vi "ExecuteCommand.vi"(11 "Command":string) -> ()   [LabVIEW 2015]
uses:
  <vilib>/Rock Robotics/Network Tables/SD Write String.vi
panel:
  out "array w/ subset deleted":string[](array[string])
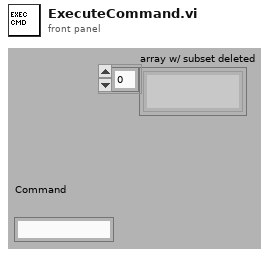
[diagram p1: front panel]
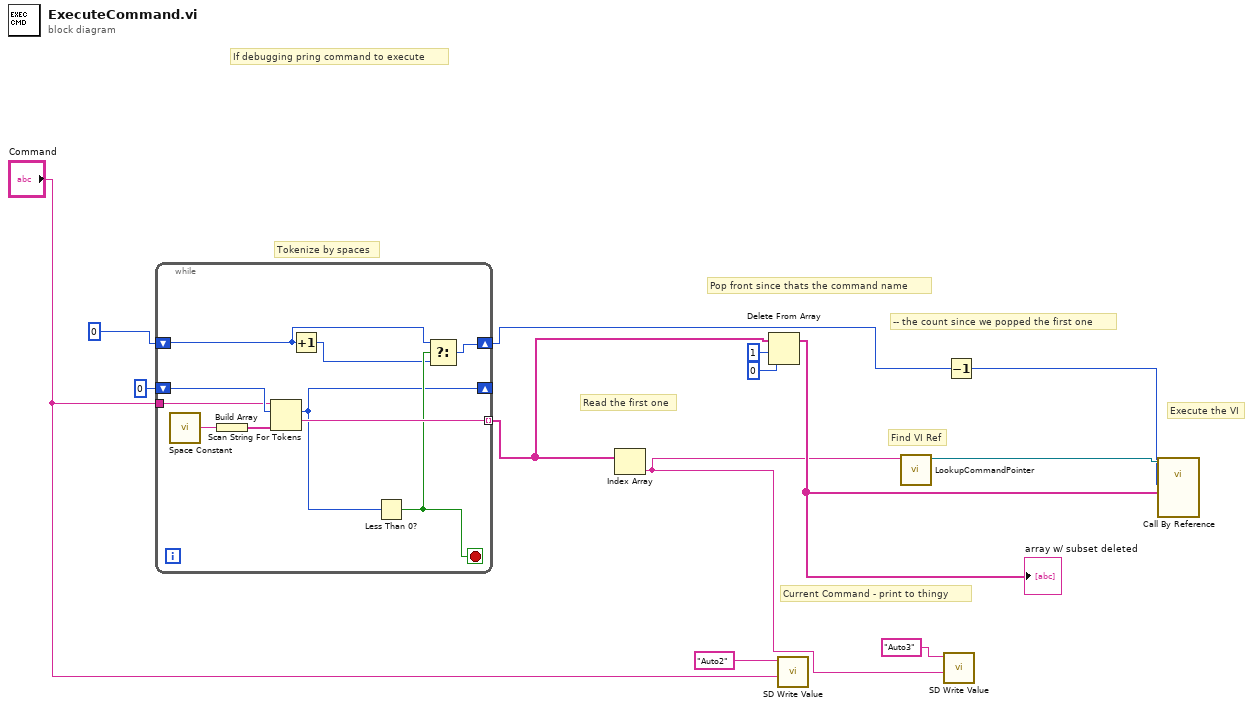
[diagram p0: block diagram]
diagram:
  # "Current Command - print to thingy"
  # "If debugging pring command to execute"
  # "Execute the VI"
  # "-- the count since we popped the first one"
  # "Pop front since thats the command name"
  # "Find VI Ref"
  # "Read the first one"
  # "Tokenize by spaces"
  n1 = while {
    shift-right: [w14] -> _
    shift-left: 0 ("offset past token") -> [w23]
    tunnel: "Command" -> [w22]
    tunnel: [w21] -> w7 mode=indexing
    shift-right: [w17] -> w10
    shift-left: u8 0 -> [w19]
    stop <- w20 stop-if-true
    n2 = call <vilib>:"Space Constant.vi"() -> ("String"=w16:string)
    n3 = Build Array(w16) -> (w15:string[])
    n4 = Scan String For Tokens(6:w15, 8:w23, 9:w22) -> (1:w21:string, 2:w14:i32)  [unwired: 5 out]
    n5 = Increment(x=w19) -> (x+1=w18:u8)
    n6 = Less Than 0?(x=w14) -> (x < 0?=w20:bool)
    n7 = Select(t=w19, s=w20, f=w18) -> (s? t:f=w17:u8)
  }
  n8 = Index Array(array=w7) -> (element=w3:string)  [unwired: 1 in]
  n9 = Delete From Array(array=w7, length=1, index=0) -> (array with subset deleted=w5:string[])  [unwired: 1 out]
  "array w/ subset deleted" <- w5
  n10 = call-poly <vilib>:"SD Write Value.vi"("String"="Command", "Name"="Auto2") -> ()  [unwired: 8 in, 2 out]
  n11 = call "LookupCommandPointer.vi"("refnum name"=w3) -> ("VI Refnum Out"=w9:refnum<vi>)  [unwired: 10 out]
  n12 = call-poly <vilib>:"SD Write Value.vi"("String"=w3, "Name"="Auto3") -> ()  [unwired: 8 in, 2 out]
  n13 = Decrement(x=w10) -> (x-1=w8:u8)
  n14 = call-by-ref "?"(reference=w9, "argv"=w5, "args"=w8) -> ()  [unwired: 11 in, 2 out]
